vi "Get Property.vi"(10 "Ctl Ref":refnum<vi>, 11 "Disabled UIP In":refnum<class "DisabledUIP.lvclass">) -> (0 "Error Out":errorcluster, 3 "Disabled UIP Out":refnum<class "DisabledUIP.lvclass">)   [LabVIEW 2015, in "DisabledUIP.lvclass"]
uses:
  DisabledUIP.lvclass
  DisabledUIP.lvclass/DisabledUIP.ctl
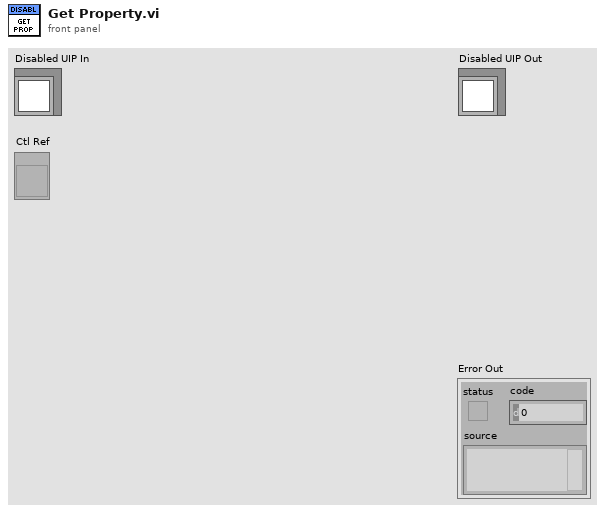
[diagram p1: front panel]
types:
  T1 = enum8{"Enabled", "Disabled", "Disabled and Grayed Out"}
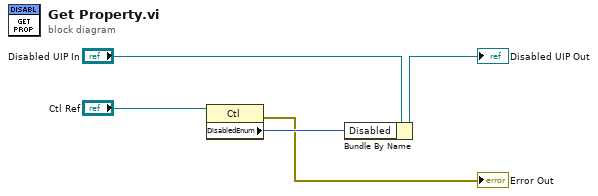
[diagram p0: block diagram]
diagram:
  n1 = property class="Ctl"(reference="Ctl Ref") -> (error out=→"Error Out":errorcluster, "DisabledEnum"=w2:T1)  [unwired: 1 in, 1 out]
  n2 = Bundle By Name(cluster="Disabled UIP In", "Disabled"=w2) -> (→"Disabled UIP Out":refnum<class "DisabledUIP.lvclass">)
